vi "Fastlite5216_ErrorCodes&Descs.vi"() -> (0 "AV_ErrorsDescs_Trans":T1(array[cluster])=[{"Code"=31000, "Name"="unknown", "Description"="unknown"}, {"Code"=31001, "Name"="invalid parameter", "Description"="invalid parameter"}, {"Code"=31002, "Name"="invalid password", "Description"="invalid password"}, {"Code"=31003, "Name"="invalid command", "Description"="invalid command"}, {"Code"=31004, "Name"="invalid size", "Description"="invalid size"}, {"Code"=31005, "Name"="meas pending", "Description"="meas pending"}, {"Code"=31006, "Name"="invalid pixel range", "Description"="invalid pixel range"}, {"Code"=31007, "Name"="invalid int. time", "Description"="invalid int. time"}, {"Code"=31008, "Name"="operation not supported", "Description"="operation not supported"}, {"Code"=31009, "Name"="invalid combination", "Description"="invalid combination"}, {"Code"=31010, "Name"="no buffer available", "Description"="no buffer available"}, {"Code"=31011, "Name"="no spectra available", "Description"="no spectra available"}, {"Code"=31012, "Name"="invalid state", "Description"="invalid state"}, {"Code"=31013, "Name"="unexpected dma int", "Description"="unexpected dma int"}, {"Code"=31014, "Name"="invalid fpga file", "Description"="invalid fpga file"}, {"Code"=31252, "Name"="invalid firmware", "Description"="Detected firmware revisions are not compatible with the driver"}, {"Code"=31253, "Name"="spectrometer not found", "Description"="cannot detect any compatible spectrometer"}, {"Code"=31254, "Name"="timeout", "Description"="timeout"}, {"Code"=31255, "Name"="unexpected response", "Description"="unexpected response"}] caption="Error Descriptions (Translated Codes)")   [LabVIEW 2012]
uses:
  Fastlite5216-VIs.lvlib
panel:
  out "Error Reason":u8(ring) format="x%02x" items=["unknown"=0, "invalid parameter"=1, "invalid password"=2, "invalid command"=3, "invalid size"=4, "meas pending"=5, "invalid pixel range"=6, "invalid int. time"=7, "operation not supported"=8, "invalid combination"=9, "no buffer available"=10, "no spectra available"=11, "invalid state"=12, "unexpected dma int"=13, "invalid fpga file"=14, "invalid firmware"=252, "spectrometer not found"=253, "timeout"=254, "unexpected response"=255]
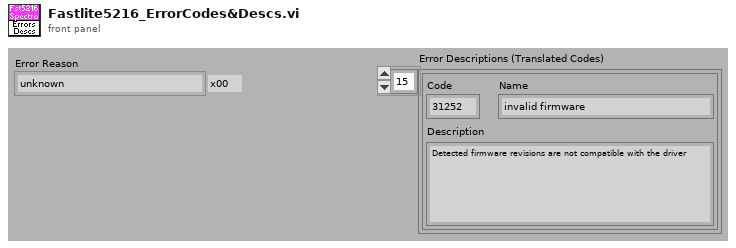
[diagram p1: front panel]
types:
  T1 = cluster{"Code":i32, "Name":string, "Description":string}[]
  T2 = cluster{"Code":i32, "Name":string, "Description":string}
  T3 = typedef "LVStringsAndValuesArrayTypeDef_U8.ctl" = cluster{"String":string, "Value":u8}[]
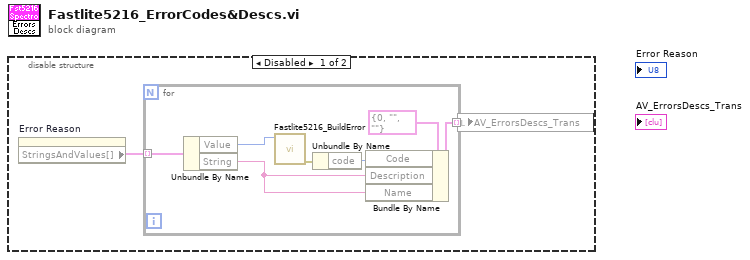
[diagram p0: block diagram]
diagram:
  n1 = disable-structure shown="Disabled" {
    frame Disabled {
      n2 = property on="Error Reason" class="Ring (strict)"() -> ("StringsAndValues[]"=w2:T3)  [unwired: 2 in, 2 out]
      n3 = for {
        tunnel: w2 -> [w7] mode=indexing
        tunnel: [w5] -> w1 mode=indexing
        n4 = Unbundle By Name(w7) -> ("Value"=w9:u8, "String"=w3:string)
        n5 = call "Fastlite5216_BuildError.vi"("Error Reason"=w9) -> ("error out"=w8:errorcluster)  [unwired: 10 in]
        n6 = Unbundle By Name(w8) -> ("code"=w6:i32)
        n7 = Bundle By Name(cluster=T2 {"Code"=0, "Name"="", "Description"=""} ("Cluster"), "Code"=w6, "Description"=w3, "Name"=w3) -> (w5:T2)
      }
      n8 = local write "AV_ErrorsDescs_Trans"(w1) -> ()
    }
    frame Enabled {
    }
  }
